vi "Transmit Data to Subscriber.vi"(8 "error in (no error)":errorcluster, 10 "Received Data":string, 11 "WebSocket Service Actor in":refnum<class "WebSocket Service Actor.lvclass">) -> (0 "error out":errorcluster, 3 "WebSocket Service Actor out":refnum<class "WebSocket Service Actor.lvclass">)   [LabVIEW 2016, in "WebSocket Actor.lvlib" / "WebSocket Service Actor.lvclass"]
uses:
  WebSocket Service Actor.lvclass
  WebSocket Service Actor.lvclass/WebSocket Service Actor.ctl
  Abstract Messages/WebSocket Data Handler Msg/WebSocket Data Handler Msg.lvclass/WebSocket Data Handler Msg.ctl
  <vilib>/ActorFramework/Message Enqueuer/Message Enqueuer.lvclass/Message Enqueuer.ctl
  <vilib>/ActorFramework/Message Enqueuer/Enqueue.vi
  Abstract Messages/WebSocket Data Handler Msg/WebSocket Data Handler Msg.lvclass
  C:/Program Files (x86)/National Instruments/LabVIEW 2016/vi.lib/ActorFramework/Message/Message.lvclass
  <vilib>/ActorFramework/Message Priority Queue/Priority Enqueue.vi
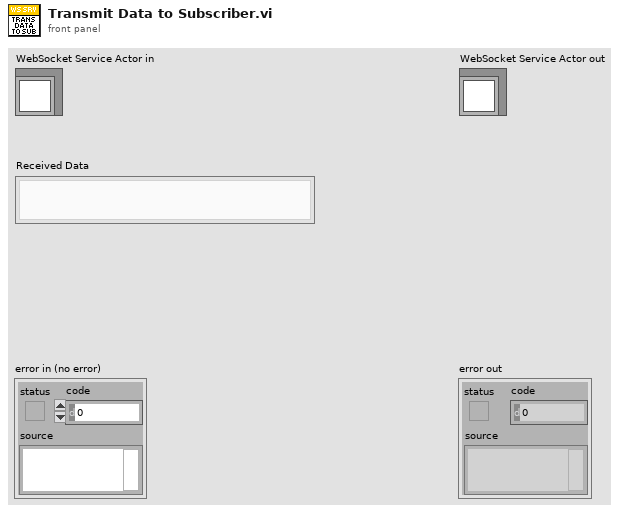
[diagram p1: front panel]
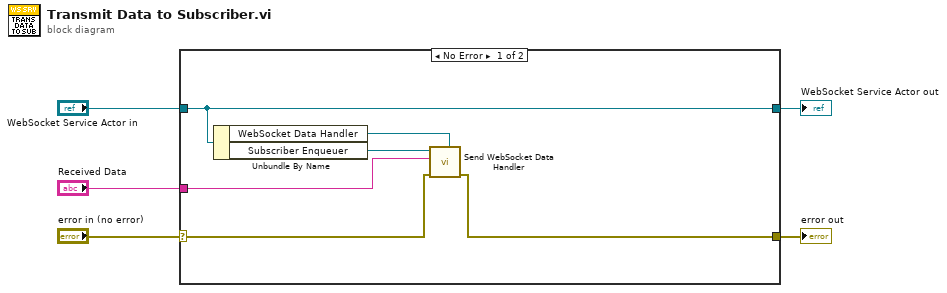
[diagram p0: block diagram]
diagram:
  n1 = case shown="No Error" "error in (no error)" {
    selector: "error in (no error)" -> [w8 w13]
    tunnel: [w7 w13] -> w4
    tunnel: [w11 w12] -> w2
    tunnel: "WebSocket Service Actor in" -> [w11 w12]
    tunnel: "Received Data" -> [w6 _]
    frame No Error {
      n2 = Unbundle By Name(w11) -> ("WebSocket Data Handler"=w9:refnum<class "WebSocket Data Handler Msg.lvclass">, "Subscriber Enqueuer"=w10:refnum<class "Message Enqueuer.lvclass">)
      n3 = call "Send WebSocket Data Handler.vi"("Message Type"=w9, "error in (no error)"=w8, "Data"=w6, "Message Enqueuer"=w10) -> ("error out"=w7:errorcluster)  [unwired: 6 in, 1 out]
    }
    frame Error {
    }
  }
  "error out" <- w4
  "WebSocket Service Actor out" <- w2
